vi "Launch Central System.vi"   [LabVIEW 2021]
uses:
  Central Control/Central Control.lvclass
  C:/Program Files (x86)/National Instruments/LabVIEW 2021/vi.lib/ActorFramework/Actor/Actor.lvclass
  <vilib>/ActorFramework/Actor/Actor.lvclass
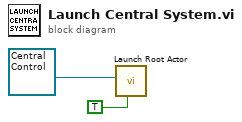
[diagram p0: block diagram]
diagram:
  n1 = call <vilib>:"Launch Root Actor.vi"("Open Actor Core front panel? (F)"=TRUE, "Actor"=refnum<class "Central Control.lvclass"> refnum ("Central Control.lvlib:Central Control.lvclass")) -> ()  [unwired: 8 in, 2 out]
